vi "FG JAUS Go.vi"(1 "FG Action (Read)":T1, 2 "Go In":bool) -> (0 "Go Out":bool)   [LabVIEW 2009]
uses:
  cRIO/Functional Global Variables/Actions for FG's.ctl
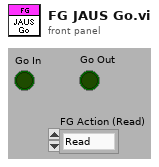
[diagram p1: front panel]
types:
  T1 = typedef "Actions for FG's.ctl" = enum16{"Read", "Write"}
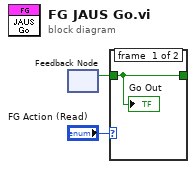
[diagram p0: block diagram]
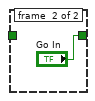
[diagram p2: hidden frame]
diagram:
  n1 = feedback #1() -> (w1:bool)  [unwired: 1 in]
  n2 = case shown="\"Read\", Default" "FG Action (Read)" {
    tunnel: w1 -> [w4 _]
    tunnel: [w4 "Go In"] -> w3
    frame #0 {
      "Go Out" <- w4
    }
    frame #1 {
    }
  }
